vi "WinPositioner_v23.vi"(0 "Display?":bool, 3 "Reverse":bool=TRUE, 4 "Yoffset 2":dbl, 6 "Xoffset":dbl, 7 "Image":T1, 8 "Y position":dbl(slide) scale=0.0..10.0, 9 "Fine Y position":dbl(slide) scale=0.0..10.0, 10 "Fine X position":dbl(slide) scale=0.0..10.0, 11 "X position":dbl(slide) scale=0.0..10.0) -> (1 "Y position":dbl, 2 "X position":dbl, 5 "CGH_x":T1(plugin-control))   [LabVIEW 2022 SP3]
uses:
  <vilib>/vision/Image Controls.llb/IMAQ Image.ctl
panel:
  # "1"
  # "2"
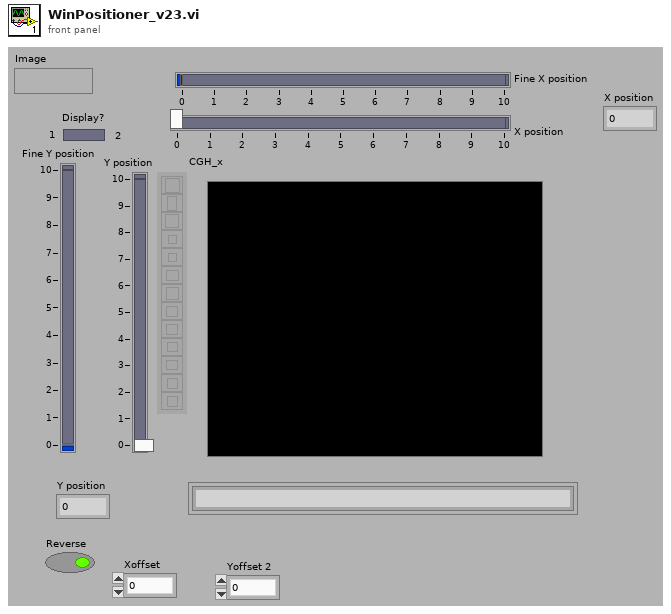
[diagram p1: front panel]
types:
  T1 = typedef "IMAQ Image.ctl" = refnum<image>
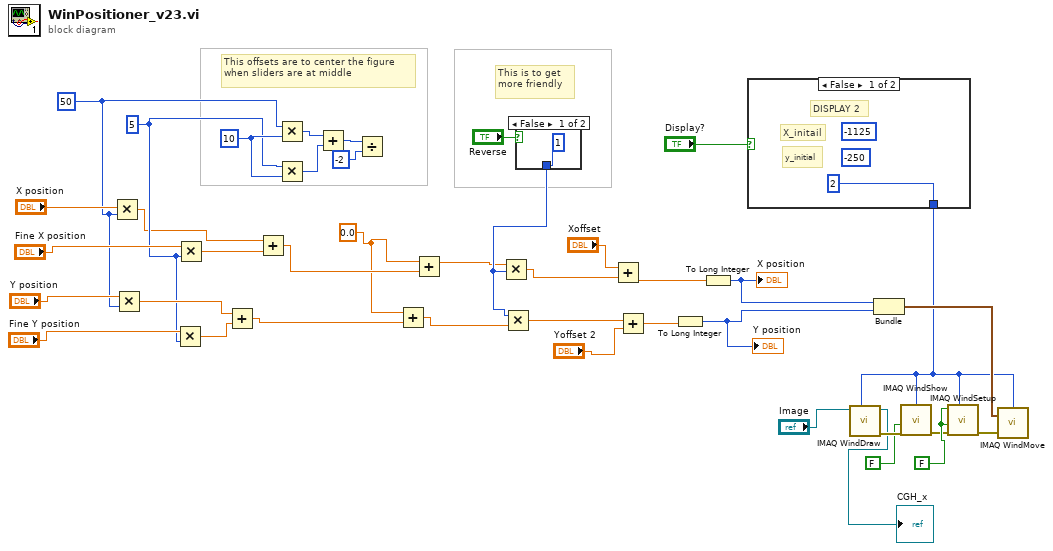
[diagram p0: block diagram]
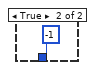
[diagram p2: hidden frame]
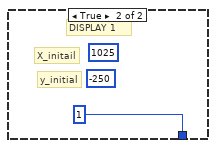
[diagram p3: hidden frame]
diagram:
  w2 = 0.0 ("x")
  w27 = 10 ("y")
  w26 = 5
  w28 = 50
  w40 = FALSE
  # "This is to get more friendly"
  # "This offsets are to center the figure when sliders are at middle"
  n1 = Multiply(x="X position", y=w28) -> (x*y=w20:dbl)
  n2 = Multiply(x="Y position", y=w28) -> (x*y=w32:dbl)
  n3 = Multiply(x="Fine Y position", y=w26) -> (x*y=w31:dbl)
  n4 = Multiply(x="Fine X position", y=w26) -> (x*y=w19:dbl)
  n5 = Add(x=w32, y=w31) -> (x+y=w16:dbl)
  n6 = Add(x=w20, y=w19) -> (x+y=w17:dbl)
  n7 = Multiply(x=w28, y=w27) -> (x*y=w25:i32)
  n8 = Multiply(x=w26, y=w27) -> (x*y=w24:i32)
  n9 = Add(x=w25, y=w24) -> (x+y=w23:i32)
  n10 = Divide(x=w23, y=-2) -> ()  [unwired: 1 out]
  n11 = Add(x=w2, y=w16) -> (x+y=w13:dbl)
  n12 = Add(x=w2, y=w17) -> (x+y=w14:dbl)
  n13 = case shown="False" "Reverse" {
    tunnel: [1 ("y") -1 ("y")] -> w15
    frame False {
    }
    frame True {
    }
  }
  n14 = Multiply(x=w14, y=w15) -> (x*y=w11:dbl)
  n15 = Multiply(x=w15, y=w13) -> (x*y=w10:dbl)
  n16 = Add(x="Xoffset", y=w11) -> (x+y=w21:dbl)
  n17 = Add(x=w10, y="Yoffset 2") -> (x+y=w4:dbl)
  n18 = To Long Integer(number=w4) -> (32bit integer=w3:i32)
  "Y position" <- w3
  n19 = To Long Integer(number=w21) -> (32bit integer=w5:i32)
  "X position" <- w5
  n20 = case shown="False" "Display?" {
    tunnel: [2 1] -> w8
    frame False {
      (unwired) -250
      (unwired) -1125
      # "DISPLAY 2"
      # "y_initial"
      # "X_initail"
    }
    frame True {
      (unwired) -250
      (unwired) 1025
      # "DISPLAY 1"
      # "y_initial"
      # "X_initail"
    }
  }
  n21 = call "IMAQ WindDraw"("Window Number (0...15)"=w8, "Image"="Image") -> ("error out"=w37:errorcluster, "Image Out (duplicate)"=→"CGH_x":T1)  [unwired: 8 in]
  n22 = Bundle(w5, w3) -> (w29:cluster{i32, i32})  [unwired: 1 in]
  n23 = call "IMAQ WindShow"("error in (no error)"=w37, "Bring To Front? (N)"=FALSE, "Window Number (0...15)"=w8) -> ("error out"=w38:errorcluster)  [unwired: 3 in, 2 out]
  n24 = call "IMAQ WindSetup"("Window Number (0...15)"=w8, "error in (no error)"=w38, "Window has title bar? (Yes)"=w40, "Window can grow? (Yes)"=w40) -> ("error out"=w39:errorcluster)  [unwired: 7 in]
  n25 = call "IMAQ WindMove"("Window Number (0...15)"=w8, "Coordinates (screen)"=w29, "error in (no error)"=w39) -> ()  [unwired: 2 in, 2 out]
